vi "(误差)根号-1实部为零.vi"() -> ()   [LabVIEW 2020]
panel:
  out "=6.12303E-17":dbl
  out "r,=False":bool=TRUE
  out "theta,=True":bool=TRUE
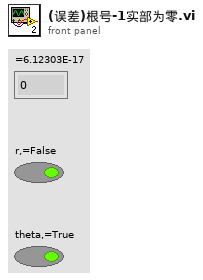
[diagram p1: front panel]
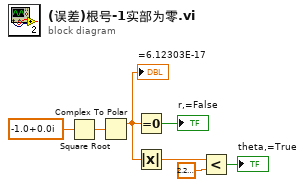
[diagram p0: block diagram]
diagram:
  n1 = Square Root(x=cdb -1.0+0.0i) -> (sqrt(x)=w6:cdb)
  n2 = Complex To Polar(r * e^(i*theta)=w6) -> (r=w1:dbl)  [unwired: 1 out]
  "=6.12303E-17" <- w1
  n3 = Equal To 0?(x=w1) -> (x = 0?=→"r,=False":bool)
  n4 = Absolute Value(x=w1) -> (abs(x)=w5:dbl)
  n5 = Less?(x=w5, y=2.220446049250313e-16) -> (x < y?=→"theta,=True":bool)
